vi "LauncherTest.vi"(8 "error in (no error)":errorcluster, 10 "SequncePath":string, 11 "TestEngine in":refnum<class "TestEngine.lvclass">) -> (0 "error out":errorcluster, 3 "TestEngine out":refnum<class "TestEngine.lvclass">)   [LabVIEW 2019, in "TestEngine.lvlib" / "TestEngine.lvclass"]
uses:
  TestEngine.lvclass
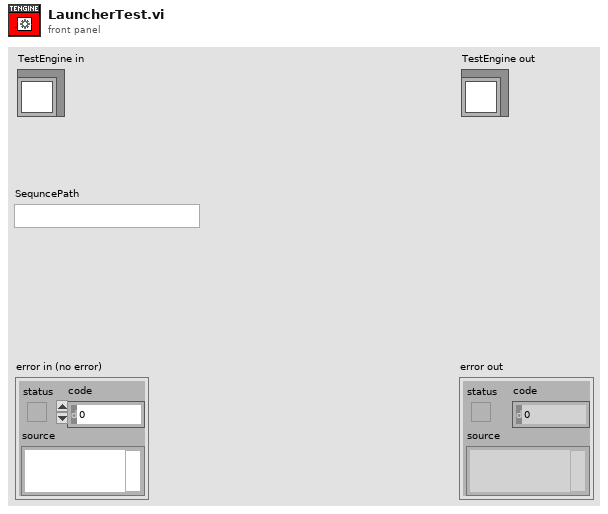
[diagram p1: front panel]
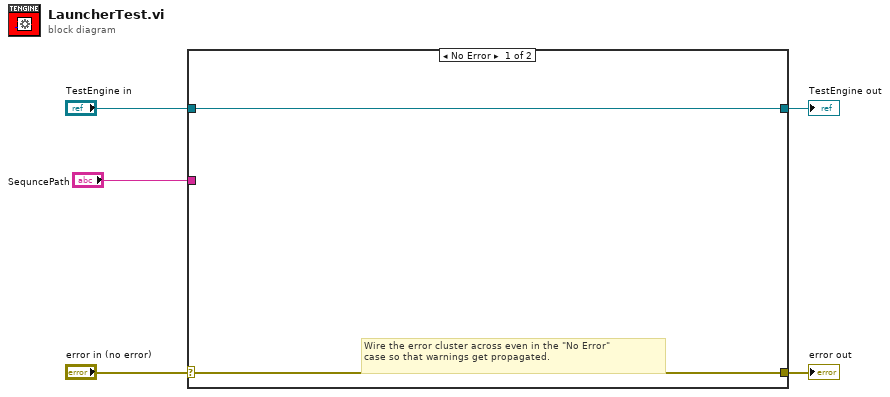
[diagram p0: block diagram]
diagram:
  n1 = case shown="No Error" "error in (no error)" {
    selector: "error in (no error)" -> [w6 w9]
    tunnel: [w6 w9] -> w4
    tunnel: [w7 w8] -> w2
    tunnel: "TestEngine in" -> [w7 w8]
    tunnel: "SequncePath" -> [_ _]
    frame No Error {
      # "Wire the error cluster across even in the \"No Error\"\ncase so that warnings get propagated."
    }
    frame Error {
    }
  }
  "error out" <- w4
  "TestEngine out" <- w2
